vi "niFPGA FFT Outside SCTL Control Unit.vi"(0 "Execution Constants":T1={"N/2-1"=7, "(N/2)*K + 1"=34, "N-1"=15, "total latency"=2, "K - 1"=3, "K - 16"=0, "K - 17"=0}, 5 "reset":bool, 7 "iteration":fxp<+,3,3>) -> (4 "control signals out":T2, 10 "stop":bool, 13 "output valid":bool, 14 "data index":u16)   [LabVIEW 2017]
uses:
  <vilib>/rvi/Analysis/measure/FFT/templates/niFPGA FFT Outside SCTL Control Signals.ctl
  <vilib>/rvi/Analysis/measure/FFT/templates/niFPGA FFT Outside SCTL States.ctl
panel:
  in  "control signals type def":T2
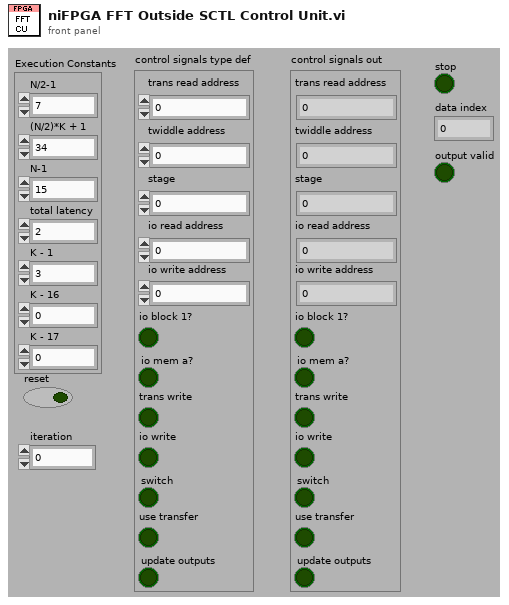
[diagram p1: front panel]
types:
  T1 = cluster{"N/2-1":u16, "(N/2)*K + 1":u16, "N-1":u16, "total latency":u16, "K - 1":u8, "K - 16":i8, "K - 17":i8}
  T2 = typedef "niFPGA FFT Outside SCTL Control Signals.ctl" = cluster{"switch":bool, "twiddle address":u16, "stage":u8, "io read address":u16, "io block 1?":bool, "trans write":bool, "io write address":u16, "update outputs":bool, "use transfer":bool, "io mem a?":bool, "io write":bool, "trans read address":u16}
  T3 = typedef "niFPGA FFT Outside SCTL States.ctl" = enum16{"Transform", "Idle"}
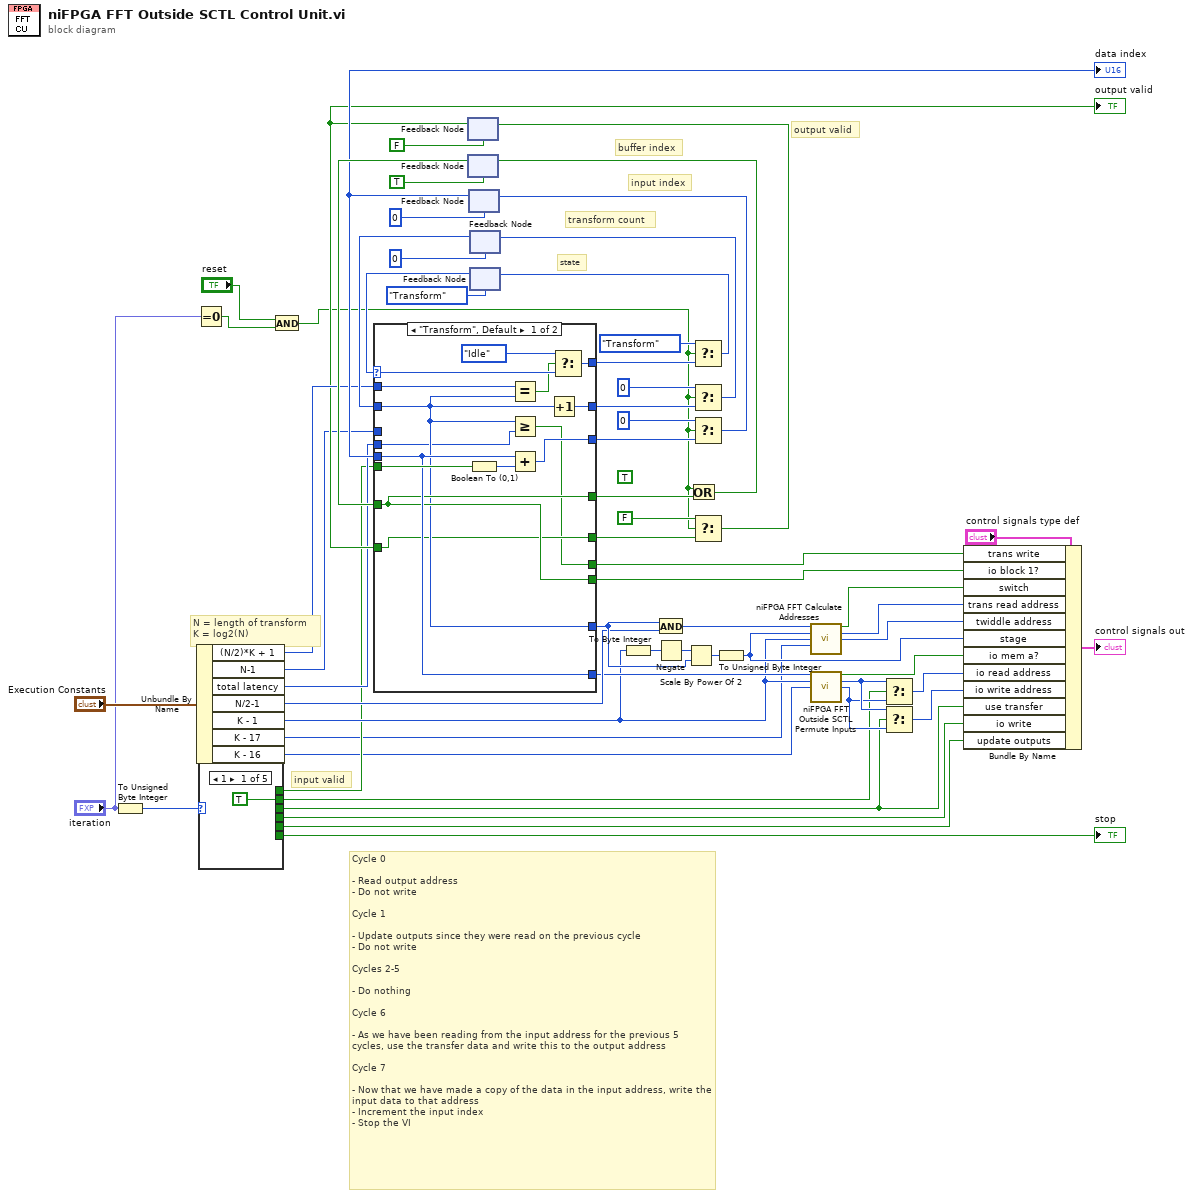
[diagram p0: block diagram]
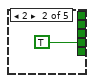
[diagram p2: hidden frame]
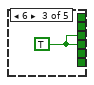
[diagram p3: hidden frame]
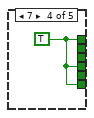
[diagram p4: hidden frame]
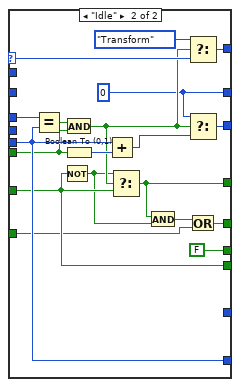
[diagram p6: hidden frame]
diagram:
  (unwired) TRUE
  # "buffer index"
  # "output valid"
  # "input index"
  # "transform count"
  # "state"
  # "input valid"
  # "Cycle 0\n\n- Read output address\n- Do not write\n\nCycle 1\n\n- Update outputs since they were read on the previous cycle\n- Do not write\n\nCycles 2-5\n\n- Do nothing\n\nCycle 6\n\n- As we have been reading from the input address for the previous 5 cycles, use the transfer data and write this to the output address\n\nCycle 7\n\n- Now that we have made a copy of the data in the input address, write the input data to that address\n- Increment the input index\n- Stop the VI"
  # "N = length of transform\nK = log2(N)"
  n1 = To Unsigned Byte Integer(number="iteration") -> (unsigned 8bit integer=w8:u8)
  n2 = Equal To 0?(x="iteration") -> (x = 0?=w11:bool)
  n3 = Unbundle By Name("Execution Constants") -> ("(N/2)*K + 1"=w41:u16, "N-1"=w31:u16, "total latency"=w35:u16, "N/2-1"=w29:u16, "K - 1"=w25:u8, "K - 17"=w1:i8, "K - 16"=w2:i8)
  n4 = case shown="1" w8 {
    tunnel: [TRUE ("x = 0?") _ _ _ _] -> w22
    tunnel: [_ _ w65 _ _] -> w10
    tunnel: [_ TRUE ("x = 0?") _ _ _] -> w14
    tunnel: [_ _ _ w66 _] -> w21
    tunnel: [_ _ _ w66 _] -> w20
    tunnel: [_ _ w65 w66 _] -> w15
    frame 1 {
    }
    frame 2 {
    }
    frame 6 {
      w65 = TRUE ("x = 0?")
    }
    frame 7 {
      w66 = TRUE
    }
    frame Default {
    }
  }
  "stop" <- w20
  n5 = And(x="reset", y=w11) -> (x .and. y?=w3:bool)
  n6 = feedback #1(FALSE) -> (w37:bool)
  "output valid" <- w37
  n7 = feedback #2(TRUE) -> (w46:bool)
  n8 = feedback #3(u16 0 ("t")) -> (w42:u16)
  "data index" <- w42
  n9 = feedback #4(u16 0 ("t")) -> (w49:u16)
  n10 = feedback #5(niFPGA_FFT_Outside_SCTL_States."Transform" ("Enum")) -> (w55:T3)
  n11 = case shown="\"Transform\", Default" w55 {
    selector: w55 -> [w79 w100]
    tunnel: w49 -> [w72 _]
    tunnel: [w81 w90] -> w54
    tunnel: w42 -> [w74 w99]
    tunnel: [w77 w89] -> w52
    tunnel: [w68 FALSE] -> w43
    tunnel: [w74 w99] -> w26
    tunnel: [w72 _] -> w30
    tunnel: w41 -> [w67 _]
    tunnel: w31 -> [_ w98]
    tunnel: [w80 w96] -> w48
    tunnel: w21 -> [w76 w85]
    tunnel: w46 -> [w73 w93]
    tunnel: [w73 w88] -> w6
    tunnel: [w73 w93] -> w45
    tunnel: [w71 w82] -> w38
    tunnel: w37 -> [w71 w83]
    tunnel: w35 -> [w70 _]
    frame "Transform", Default {
      n12 = Boolean To (0,1)(Boolean=w76) -> (0, 1=w75:i16)
      n13 = Equal?(x=w67, y=w72) -> (x = y?=w78:bool)
      n14 = Greater Or Equal?(x=w72, y=w70) -> (x >= y?=w68:bool)
      n15 = Add(x=w74, y=w75) -> (x+y=w77:u16)
      n16 = Increment(x=w72) -> (x+1=w81:u16)
      n17 = Select(t=niFPGA_FFT_Outside_SCTL_States."Idle" ("Enum"), s=w78, f=w79) -> (s? t:f=w80:T3)
    }
    frame "Idle" {
      w90 = u16 0 ("t")
      n18 = Equal?(x=w98, y=w99) -> (x = y?=w94:bool)
      n19 = Not(x=w93) -> (.not. x?=w87:bool)
      n20 = And(x=w94, y=w85) -> (x .and. y?=w91:bool)
      n21 = Boolean To (0,1)(Boolean=w85) -> (0, 1=w95:i16)
      n22 = Add(x=w99, y=w95) -> (x+y=w92:u16)
      n23 = Select(t=w87, s=w91, f=w93) -> (s? t:f=w88:bool)
      n24 = And(x=w88, y=w87) -> (x .and. y?=w84:bool)
      n25 = Select(t=niFPGA_FFT_Outside_SCTL_States."Transform" ("Enum"), s=w91, f=w100) -> (s? t:f=w96:T3)
      n26 = Select(t=w90, s=w91, f=w92) -> (s? t:f=w89:u16)
      n27 = Or(x=w84, y=w83) -> (x .or. y?=w82:bool)
    }
  }
  n28 = To Byte Integer(number=w25) -> (8bit integer=w32:i8)
  n29 = And(x=w30, y=w29) -> (x .and. y?=w28:u16)
  n30 = Negate(x=w32) -> (-x=w34:i8)
  n31 = Scale By Power Of 2(n=w34, x=w30) -> (x*2^n=w33:u16)
  n32 = Or(x=w3, y=w6) -> (x .or. y?=w5:bool)
  n33 = feedback-in #2(w5) -> ()
  n34 = Select(t=niFPGA_FFT_Outside_SCTL_States."Transform" ("Enum"), s=w3, f=w48) -> (s? t:f=w58:T3)
  n35 = feedback-in #5(w58) -> ()
  n36 = Select(t=u16 0, s=w3, f=w54) -> (s? t:f=w56:u16)
  n37 = feedback-in #4(w56) -> ()
  n38 = Select(t=u16 0, s=w3, f=w52) -> (s? t:f=w57:u16)
  n39 = feedback-in #3(w57) -> ()
  n40 = Select(t=FALSE, s=w3, f=w38) -> (s? t:f=w7:bool)
  n41 = feedback-in #1(w7) -> ()
  n42 = To Unsigned Byte Integer(number=w33) -> (unsigned 8bit integer=w27:u8)
  n43 = call <vilib>:"niFPGA FFT Calculate Addresses.vi"("butterfly count"=w28, "current stage"=w27, "K - 1"=w25, "K - 17"=w1) -> ("switch?"=w36:bool, "address"=w62:u16, "twiddle index"=w61:u16)  [unwired: 9 out]
  n44 = call <vilib>:"niFPGA FFT Outside SCTL Permute Inputs.vi"("input index"=w26, "K - 1"=w25, "K - 16"=w2) -> ("mem block A?"=w18:bool, "output address"=w24:u16, "input address"=w23:u16)  [unwired: 10 out]
  n45 = Select(t=w24, s=w22, f=w23) -> (s? t:f=w17:u16)
  n46 = Select(t=w24, s=w10, f=w23) -> (s? t:f=w16:u16)
  n47 = Bundle By Name(cluster="control signals type def", "trans write"=w43, "io block 1?"=w45, "switch"=w36, "trans read address"=w62, "twiddle address"=w61, "stage"=w27, "io mem a?"=w18, "io read address"=w17, "io write address"=w16, "use transfer"=w10, "io write"=w15, "update outputs"=w14) -> (→"control signals out":T2)
